vi "create coeffs(subVI).vi"(9 "auto z adjust":T1, 10 "Array in":dbl[][][][](array[numeric]), 11 "config in":T2) -> (3 "Array out":dbl[][](array[numeric]))   [LabVIEW 2024]
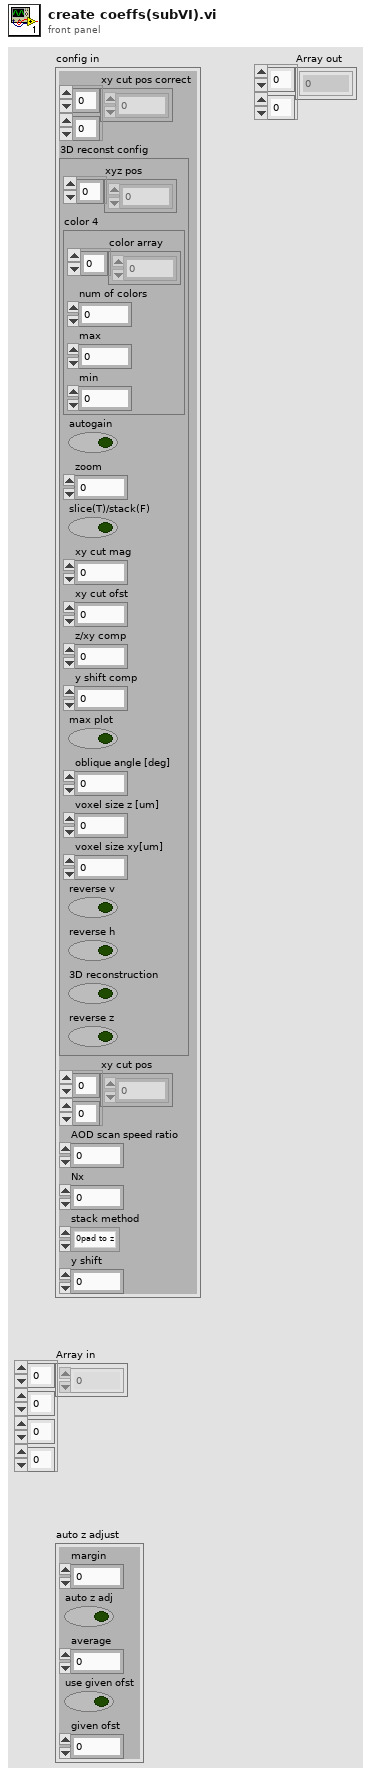
[diagram p1: front panel]
types:
  T1 = cluster{"margin":dbl, "auto z adj":bool, "average":i32, "use given ofst":bool, "given ofst":i32}
  T2 = cluster{"xy cut pos correct":dbl[][], "3D reconst config":cluster{"xyz pos":u16[], "color 4":cluster{"color array":u32[], "num of colors":i32, "max":dbl, "min":dbl}, "autogain":bool, "zoom":dbl, "slice(T)/stack(F)":bool, "xy cut mag":dbl, "xy cut ofst":dbl, "z/xy comp":dbl, "y shift comp":dbl, "max plot":bool, "oblique angle [deg]":dbl, "voxel size z [um]":dbl, "voxel size xy[um]":dbl, "reverse v":bool, "reverse h":bool, "3D reconstruction":bool, "reverse z":bool}, "xy cut pos":dbl[][], "AOD scan speed ratio":dbl, "Nx":dbl, "stack method":enum16{"0pad to z", "0pad to x", "0pad to x and rot"}, "y shift":i32}
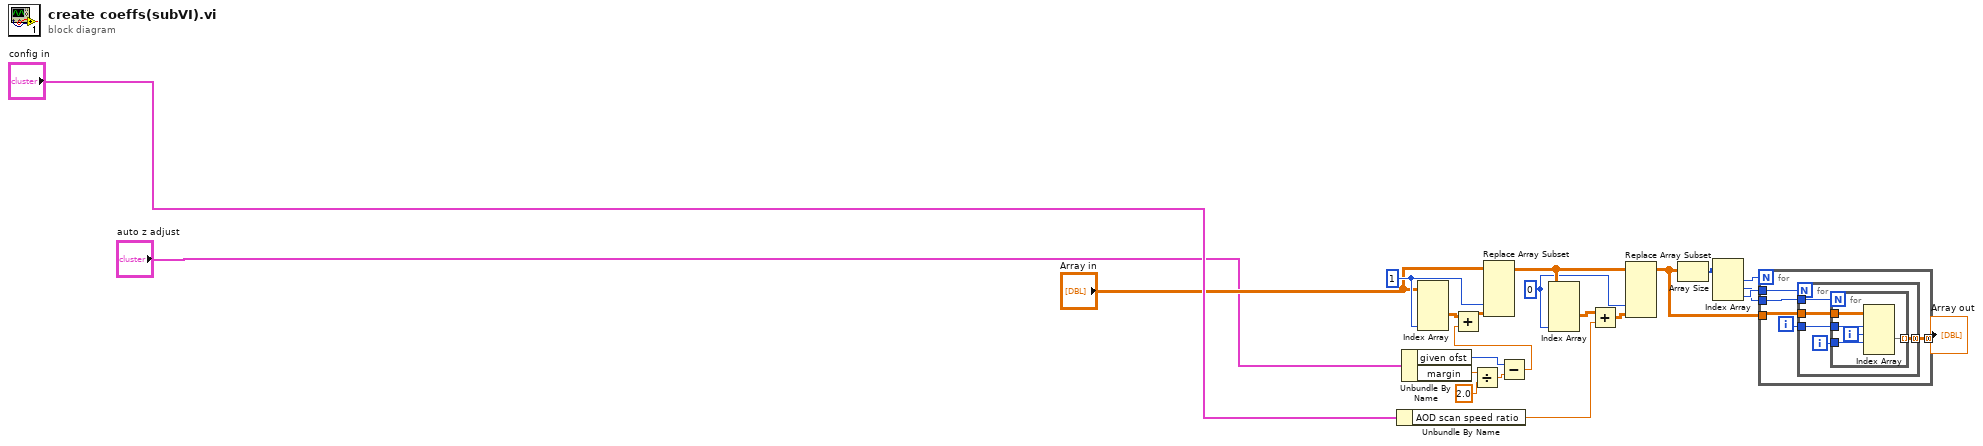
[diagram p0: block diagram]
diagram:
  w11 = 0 ("disabled index (col)")
  w10 = 1 ("disabled index (col)")
  n1 = Unbundle By Name("config in") -> ("AOD scan speed ratio"=w16:dbl)
  n2 = Unbundle By Name("auto z adjust") -> ("given ofst"=w5:i32, "margin"=w2:dbl)
  n3 = Index Array(array="Array in", index (dim 3)=w10) -> (element=w7:dbl[][][])  [unwired: 3 in]
  n4 = Divide(x=w2, y=2.0) -> (x/y=w4:dbl)
  n5 = Subtract(x=w5, y=w4) -> (x-y=w8:dbl)
  n6 = Add(x=w7, y=w8) -> (x+y=w6:dbl[][][])
  n7 = Replace Array Subset(array="Array in", new element=w6, index (dim 3)=w10) -> (w14:dbl[][][][])  [unwired: 3 in]
  n8 = Index Array(array=w14, index (dim 3)=w11) -> (element=w12:dbl[][][])  [unwired: 3 in]
  n9 = Add(x=w12, y=w16) -> (x+y=w13:dbl[][][])
  n10 = Replace Array Subset(array=w14, new element=w13, index (dim 3)=w11) -> (w21:dbl[][][][])  [unwired: 3 in]
  n11 = Array Size(array=w21) -> (size(s)=w17:i32[])
  n12 = Index Array(array=w17) -> (element #1=w18:i32, element #2=w19:i32, element #3=w20:i32)  [unwired: 3 in]
  n13 = for {
    N: w18 -> [_]
    tunnel: w21 -> [w27]
    tunnel: w19 -> [w26]
    tunnel: w20 -> [w25]
    tunnel: [w23] -> w22 mode=concatenating
    i -> [w24]
    n14 = for {
      N: w25 -> [_]
      tunnel: w27 -> [w32]
      tunnel: w26 -> [w31]
      tunnel: w24 -> [w30]
      tunnel: [w28] -> w23 mode=concatenating
      i -> [w29]
      n15 = for {
        N: w31 -> [_]
        tunnel: w32 -> [w37]
        tunnel: w30 -> [w36]
        tunnel: w29 -> [w35]
        tunnel: [w33] -> w28 mode=indexing
        i -> [w34]
        n16 = Index Array(array=w37, index (dim 0)=w36, index (dim 1)=w34, index (dim 2)=w35) -> (element=w33:dbl[])  [unwired: 1 in]
      }
    }
  }
  "Array out" <- w22
